vi "MFC_test.vi"() -> ()   [LabVIEW 2017]
panel:
  in  "Manual?":bool=TRUE
  in  "Manual Setpoint (sccm)":dbl caption="Offset" min=0.0 max=20.0 step=0.5
  out "valve close":dynamicdata(graph)=[{"t0"=timestamp(3663317035.751964 s since 1904-01-01), "dt"=5.0, "Y"=[0.0], "attributes"=variant("NI_ChannelName"=variant(string "Signal"), "NI_ExpIsRelativeTime"=variant(bool FALSE), "NI_ExpStartTimeStamp"=variant(timestamp timestamp(3663316430.751964 s since 1904-01-01)), "NI_ExpTimeStamp"=variant(timestamp timestamp(3663317130.814712 s since 1904-01-01)), "NI_ExpXDimension"=variant(string "t"))}]
  out "purge":dynamicdata(graph)=[{"t0"=timestamp(3663317035.751964 s since 1904-01-01), "dt"=5.0, "Y"=[0.0], "attributes"=variant("NI_ChannelName"=variant(string "Signal"), "NI_ExpIsRelativeTime"=variant(bool FALSE), "NI_ExpStartTimeStamp"=variant(timestamp timestamp(3663316430.751964 s since 1904-01-01)), "NI_ExpTimeStamp"=variant(timestamp timestamp(3663317130.814712 s since 1904-01-01)), "NI_ExpXDimension"=variant(string "t"))}]
  out "Setpoint":dynamicdata(graph)=[{"t0"=timestamp(3663317035.751964 s since 1904-01-01), "dt"=5.0, "Y"=[0.0], "attributes"=variant("NI_ChannelName"=variant(string "Signal"), "NI_ExpIsRelativeTime"=variant(bool FALSE), "NI_ExpStartTimeStamp"=variant(timestamp timestamp(3663316430.751964 s since 1904-01-01)), "NI_ExpTimeStamp"=variant(timestamp timestamp(3663317130.814712 s since 1904-01-01)), "NI_ExpXDimension"=variant(string "t"))}]
  in  "stop":bool
  out "sccm":dynamicdata(graph)=[{"t0"=timestamp(3663317035.751964 s since 1904-01-01), "dt"=5.0, "Y"=[0.0], "attributes"=variant("NI_ChannelName"=variant(string "Signal"), "NI_ExpIsRelativeTime"=variant(bool FALSE), "NI_ExpStartTimeStamp"=variant(timestamp timestamp(3663316430.751964 s since 1904-01-01)), "NI_ExpTimeStamp"=variant(timestamp timestamp(3663317130.814712 s since 1904-01-01)), "NI_ExpXDimension"=variant(string "t"))}]
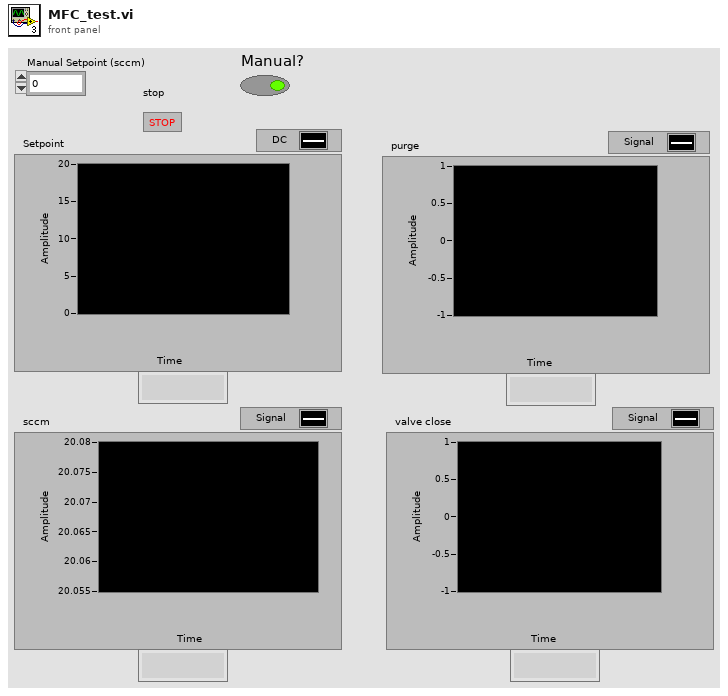
[diagram p1: front panel]
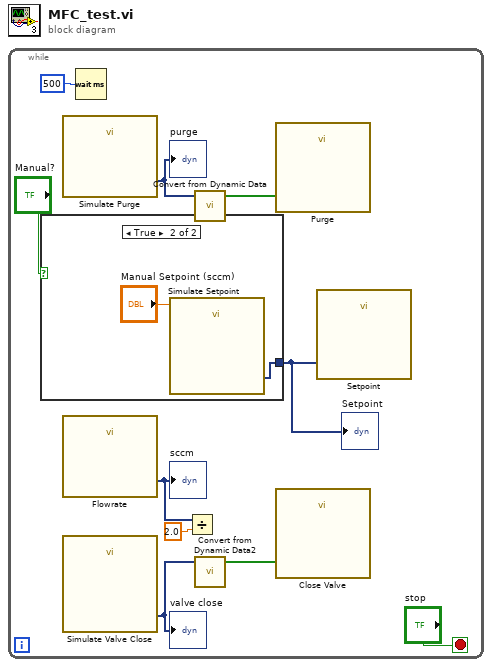
[diagram p0: block diagram]
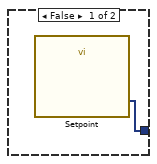
[diagram p2: hidden frame]
diagram:
  n1 = while {
    stop <- "stop" stop-if-true
    n2 = case shown="True" "Manual?" {
      tunnel: [w11 w13] -> w1
      frame False {
        n3 = call "Setpoint"() -> ("Signal"=w11:dynamicdata)  [unwired: 9 in, 2 out]
      }
      frame True {
        n4 = call "Simulate Setpoint"("Offset"="Manual Setpoint (sccm)") -> ("DC"=w13:dynamicdata)  [unwired: 13 in, 1 out]
      }
    }
    "Setpoint" <- w1
    n5 = call "Simulate Purge"() -> ("Signal"=w6:dynamicdata)  [unwired: 9 in, 2 out]
    "purge" <- w6
    n6 = call "Flowrate"() -> ("data"=w7:dynamicdata)  [unwired: 17 in, 2 out]
    "sccm" <- w7
    n7 = call "Simulate Valve Close"() -> ("Signal"=w4:dynamicdata)  [unwired: 9 in, 2 out]
    "valve close" <- w4
    n8 = Wait (ms)(milliseconds to wait=u32 500) -> ()  [unwired: 1 out]
    n9 = Divide(x=w7, y=2.0) -> ()  [unwired: 1 out]
    n10 = call "Convert from Dynamic Data"("Dynamic Data Type"=w6) -> ("Array"=w5:bool[])  [unwired: 3 in]
    n11 = call "Convert from Dynamic Data2"("Dynamic Data Type"=w4) -> ("Array"=w3:bool[])  [unwired: 3 in]
    n12 = call "Purge"("data"=w5) -> ()  [unwired: 17 in, 2 out]
    n13 = call "Close Valve"("data"=w3) -> ()  [unwired: 17 in, 2 out]
    n14 = call "Setpoint"("data"=w1) -> ()  [unwired: 17 in, 2 out]
  }
